vi "Project Tree Process Keydown Event.vi"(8 "Project Tree":refnum<vi>, 10 "Ctrl":bool, 11 "ScanCode":i16) -> (0 "Step Operation Data":T1, 2 "Operation Accept":bool, 3 "Event Discard":bool)   [LabVIEW 2015, in "Editor.lvclass"]
uses:
  Editor.lvclass
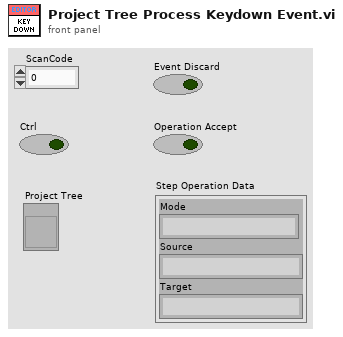
[diagram p1: front panel]
types:
  T1 = cluster{"Mode":string, "Source":string, "Target":string}
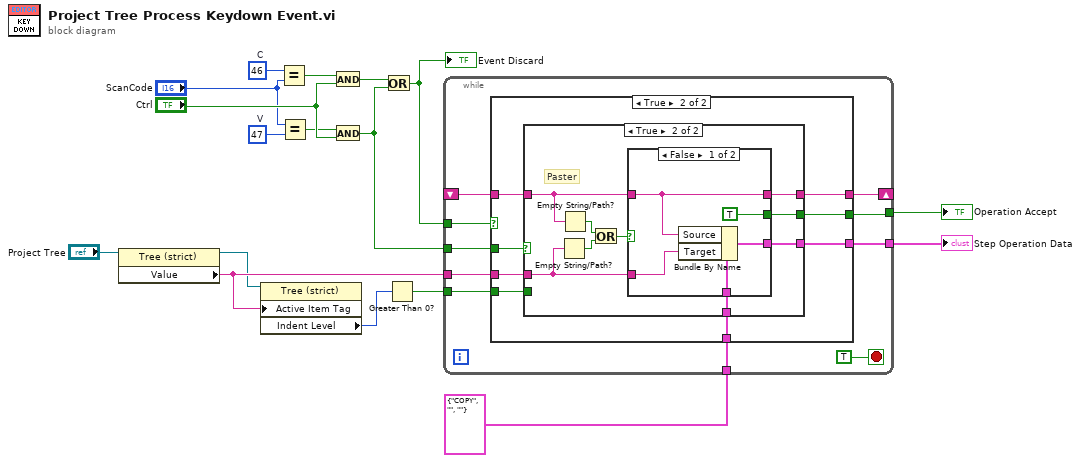
[diagram p0: block diagram]
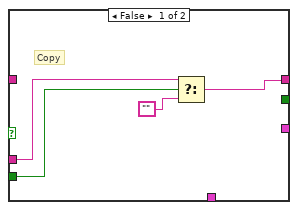
[diagram p3: hidden frame]
diagram:
  w13 = i16 47  # V
  w12 = i16 46  # C
  n1 = property class="Tree (strict)"(reference="Project Tree") -> (reference out=w2:refnum<vi>, "Value"=w3:string)  [unwired: 1 in, 1 out]
  n2 = property class="Tree (strict)"(reference=w2, "Active Item Tag"=w3) -> ("Indent Level"=w1:i32)  [unwired: 1 in, 2 out]
  n3 = Equal?(x=w12, y="ScanCode") -> (x = y?=w14:bool)
  n4 = Equal?(x="ScanCode", y=w13) -> (x = y?=w15:bool)
  n5 = And(x=w14, y="Ctrl") -> (x .and. y?=w11:bool)
  n6 = And(x=w15, y="Ctrl") -> (x .and. y?=w8:bool)
  n7 = Or(x=w11, y=w8) -> (x .or. y?=w9:bool)
  "Event Discard" <- w9
  n8 = Greater Than 0?(x=w1) -> (x > 0?=w7:bool)
  n9 = while {
    tunnel: w9 -> [w27]
    tunnel: w8 -> [w26]
    tunnel: w3 -> [w25]
    tunnel: w7 -> [w24]
    shift-right: [w22] -> _
    shift-left: _ -> [w21]
    tunnel: T1 {"Mode"="COPY", "Source"="", "Target"=""} ("Step Operation Data") -> [w20]
    tunnel: [w19] -> w5
    tunnel: [w18] -> w4
    stop <- TRUE stop-if-true
    n10 = case shown="True" w27 {
      tunnel: w26 -> [_ w36]
      tunnel: w25 -> [_ w35]
      tunnel: w24 -> [_ w34]
      tunnel: [w28 w33] -> w22
      tunnel: w21 -> [w28 w32]
      tunnel: w20 -> [_ w31]
      tunnel: [_ w30] -> w19
      tunnel: [_ w29] -> w18
      frame False {
      }
      frame True {
        n11 = case shown="True" w36 {
          tunnel: w35 -> [w39 w43]
          tunnel: w34 -> [w40 _]
          tunnel: [w37 w44] -> w33
          tunnel: w32 -> [_ w45]
          tunnel: w31 -> [_ w46]
          tunnel: [_ w42] -> w30
          tunnel: [_ w41] -> w29
          frame False {
            # "Copy"
            n12 = Select(t=w39, s=w40, f="") -> (s? t:f=w37:string)
          }
          frame True {
            # "Paster"
            n13 = Empty String/Path?(string/path=w43) -> (empty?=w49:bool)
            n14 = Empty String/Path?(string/path=w45) -> (empty?=w48:bool)
            n15 = Or(x=w48, y=w49) -> (x .or. y?=w47:bool)
            n16 = case shown="False" w47 {
              tunnel: w46 -> [w54 _]
              tunnel: w45 -> [w53 w55]
              tunnel: [w53 w55] -> w44
              tunnel: w43 -> [w52 _]
              tunnel: [w51 _] -> w42
              tunnel: [TRUE _] -> w41
              frame False {
                n17 = Bundle By Name(cluster=w54, "Source"=w53, "Target"=w52) -> (w51:T1)
              }
              frame True {
              }
            }
          }
        }
      }
    }
  }
  "Operation Accept" <- w4
  "Step Operation Data" <- w5
